vi "MasterRobotModeController.vi"() -> (1 "FMS Robot Mode":T1, 2 "Auto Reset":bool, 3 "Robot is Autonomous":bool)   [LabVIEW 2019]
doc: "This state controller manages the Robot Mode and whether or not the robot is running autonomously. The robot will continue running autonomously after Autonomous Mode ends, until the driver touches the joystick during TeleOperated Mode. The Auto Test Heading is also managed by this VI when in Auto Test Mode as set by the FRC 4265 Dashboard."
uses:
  <vilib>/Rock Robotics/WPI/DriverStation/WPI_DriverStationRobotMode2.ctl
  refnums.vi
  dsdata.vi
  GRNF_Joystick.vi
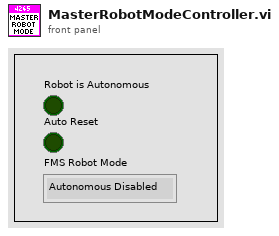
[diagram p1: front panel]
types:
  T1 = typedef "WPI_DriverStationRobotMode2.ctl" = enum16{"Autonomous Disabled", "Autonomous Enabled", "Teleop Disabled", "Teleop Enabled", "Disconnected", "Finish", "Test Disabled", "Test Enabled", "Emergency Stopped"}
  T2 = typedef "WPI_JoystickDevRef.ctl" = cluster{"Device":T3}
  T3 = typedef "WPI_JoystickDeviceEnum.ctl" = enum16{"USB 0", "USB 1", "USB 2", "USB 3", "USB 4", "USB 5"}
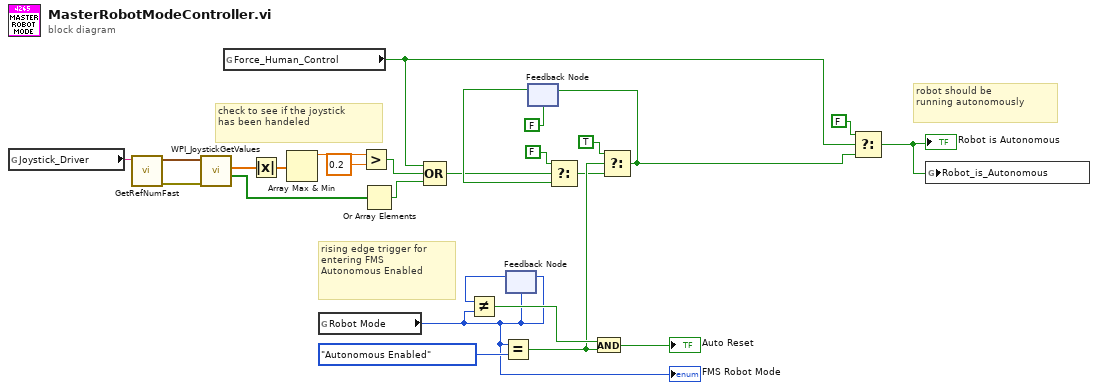
[diagram p0: block diagram]
diagram:
  # "rising edge trigger for\nentering FMS\nAutonomous Enabled"
  # "robot should be\nrunning autonomously"
  # "check to see if the joystick \nhas been handeled"
  n1 = global read "refnums.vi" "Joystick_Driver"() -> (w24:string)
  n2 = call-poly "GetRefNumFast.vi"("RefNum Name"=w24) -> ("Error"=w25:errorcluster, "Device Reference"=w26:T2)  [unwired: 5 in]
  n3 = call <vilib>:"WPI_JoystickGetValues.vi"("error in (no error)"=w25, "JoystickDevRef"=w26) -> ("Buttons"=w23:bool[], "Axes"=w22:dbl[])  [unwired: 5 in, 3 out]
  n4 = global read "dsdata.vi" "Force_Human_Control"() -> (w1:bool)
  n5 = Absolute Value(x=w22) -> (abs(x)=w21:dbl[])
  n6 = Array Max & Min(array=w21) -> (max value=w20:dbl)  [unwired: 3 out]
  n7 = global read "dsdata.vi" "Robot Mode"() -> (w5:T1)
  "FMS Robot Mode" <- w5
  n8 = Greater?(x=w20, y=0.2) -> (0:w18:bool)
  n9 = Or Array Elements(Boolean array=w23) -> (logical OR=w17:bool)
  n10 = Compound Arithmetic op=OR(w1, w18, w17) -> (w6:bool)
  n11 = Equal?(x=w5, y=WPI_DriverStationRobotMode2."Autonomous Enabled" ("Robot Mode")) -> (x = y?=w10:bool)
  n12 = feedback #1(w5) -> (w13:T1)
  n13 = Not Equal?(x=w13, y=w5) -> (x != y?=w12:bool)
  n14 = feedback-in #1(w5) -> ()
  n15 = feedback #2(FALSE) -> (w7:bool)
  n16 = Select(t=FALSE, s=w6, f=w7) -> (s? t:f=w8:bool)
  n17 = And(x=w12, y=w10) -> (x .and. y?=→"Auto Reset":bool)
  n18 = Select(t=TRUE, s=w10, f=w8) -> (s? t:f=w3:bool)
  n19 = feedback-in #2(w3) -> ()
  n20 = Select(t=FALSE, s=w1, f=w3) -> (s? t:f=w2:bool)
  "Robot is Autonomous" <- w2
  n21 = global write "dsdata.vi" "Robot_is_Autonomous"(w2) -> ()
